vi "Aurora Config.vi"(0 "6592R Resources":T1[](array[typedef]), 5 "Simulate and check Data":bool, 7 "FIFO Depth":u32=10240000 format="%#.6p", 9 "USRP RIO Resources":T1[](array[typedef]), 11 "error in (no error)":errorcluster) -> (4 "Ports used":bool[](array[boolean]), 6 "Refnum out":refnum<k20>[](array[refnum]), 10 "2 USRPs?":bool[](array[boolean]), 15 "error out":errorcluster)   [LabVIEW 2016]
uses:
  <vilib>/userdefined/Silver/nirio_resource_slv.ctl
  6592R/SubVIs/Aurora Stream (NI 6592R) (Host).lvlib
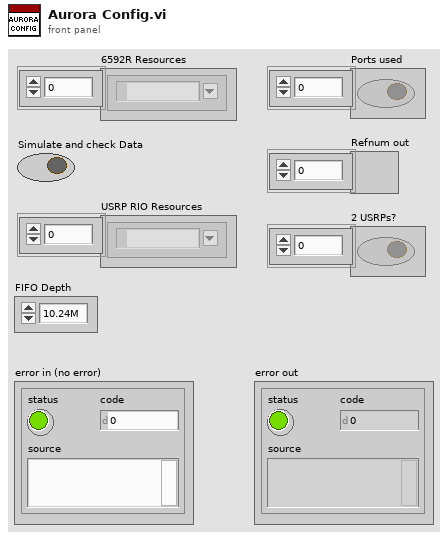
[diagram p1: front panel]
types:
  T1 = typedef "nirio_resource_slv.ctl" = tag
  T2 = cluster{"Hard Error":bool, "Soft Error":bool, "Lane Up":bool, "Channel Up":bool, "Sys Reset":bool}
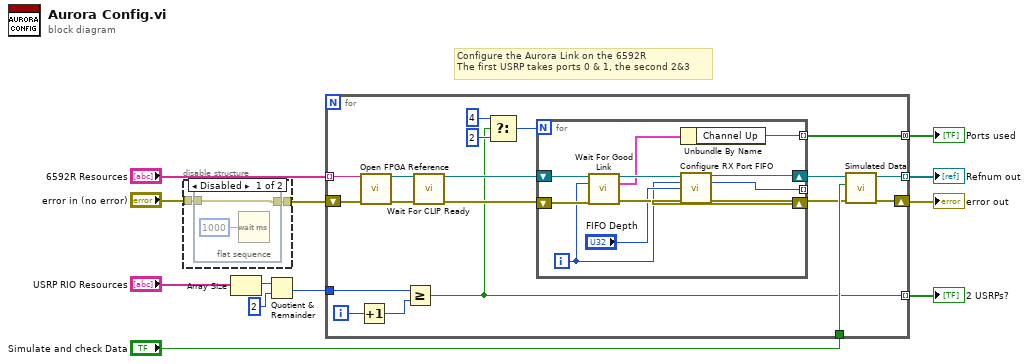
[diagram p0: block diagram]
diagram:
  # "Configure the Aurora Link on the 6592R\nThe first USRP takes ports 0 & 1, the second 2&3"
  n1 = disable-structure shown="Disabled" {
    disable-tunnel: [w14 w17] -> w9
    disable-tunnel: "error in (no error)" -> [w13 w17]
    frame Disabled {
      n2 = flat-sequence {
        tunnel: w13 -> [w16]
        tunnel: [w16] -> w14
        frame #0 {
          n3 = Wait (ms)(milliseconds to wait=u32 1000) -> ()  [unwired: 1 out]
        }
      }
    }
    frame Enabled {
    }
  }
  n4 = Array Size(array="USRP RIO Resources") -> (size(s)=w5:i32)
  n5 = Quotient & Remainder(x=w5, y=2) -> (floor(x/y)=w7:i32)  [unwired: 1 out]
  n6 = for {
    tunnel: [w29] -> w2 mode=indexing
    tunnel: "6592R Resources" -> [w34] mode=indexing
    shift-right: [w28] -> w1
    shift-left: w9 -> [w33]
    tunnel: w7 -> [w32]
    tunnel: [w18] -> w12 mode=indexing
    tunnel: "Simulate and check Data" -> [w27]
    tunnel: [w20] -> w10 mode=concatenating
    i -> [w31]
    n7 = Increment(x=w31) -> (x+1=w30:i32)
    n8 = call "Open FPGA Reference.vi"("FPGA Resource"=w34, "error in"=w33) -> ("FPGA VI Reference Out"=w35:refnum<k20>, "error out"=w36:errorcluster)  [unwired: 12 in]
    n9 = Greater Or Equal?(x=w32, y=w30) -> (x >= y?=w18:bool)
    n10 = call "Wait For CLIP Ready.vi"("Refnum in"=w35, "error in"=w36) -> ("Refnum out"=w26:refnum<k20>, "error out"=w25:errorcluster)  [unwired: 11 in, 1 out]
    n11 = Select(t=4, s=w18, f=2) -> (s? t:f=w19:i32)
    n12 = for {
      N: w19 -> [_]
      shift-right: [w43] -> w24
      shift-left: w25 -> [w47]
      shift-right: [w42] -> w23
      shift-left: w26 -> [w46]
      tunnel: [w39] -> w20 mode=indexing
      tunnel: [w37] -> _ mode=indexing
      i -> [w38]
      n13 = call "Wait For Good Link.vi"("Refnum in"=w46, "Port"=w38, "error in"=w47) -> ("Refnum out"=w44:refnum<k20>, "Port Debug Info"=w40:T2, "error out"=w45:errorcluster)  [unwired: 10 in]
      n14 = Unbundle By Name(w40) -> ("Channel Up"=w39:bool)
      n15 = call "Configure RX Port FIFO.vi"("Refnum in"=w44, "RX Port"=w38, "FIFO Depth"="FIFO Depth", "error in"=w45) -> ("Refnum out"=w42:refnum<k20>, "Actual Depth"=w37:u32, "error out"=w43:errorcluster)  [unwired: 9 in]
    }
    n16 = call "Simulated Data.vi"("error in"=w24, "Simulated Data"=w27, "Refnum in"=w23) -> ("error out"=w28:errorcluster, "Refnum out"=w29:refnum<k20>)  [unwired: 7 in]
  }
  "2 USRPs?" <- w12
  "Ports used" <- w10
  "Refnum out" <- w2
  "error out" <- w1
